vi "GetDVR.vi"(8 "error in (no error)":errorcluster, 11 "Menu in":refnum<class "Menu.lvclass">) -> (0 "error out":errorcluster, 2 "DVR":refnum<data-value>, 3 "Menu out":refnum<class "Menu.lvclass">)   [LabVIEW 2021, in "Menu.lvlib" / "Menu.lvclass"]
uses:
  Menu.lvclass
  Menu.lvclass/Menu.ctl
  MenuItems.ctl
  Data.ctl
  <vilib>/Utility/miscctls.llb/LVMenuShortCut.ctl
  MenuSelection.ctl
  TD_CloseEvent.ctl
  Picture2D/src/Color/Color.lvclass
  MenuColors.ctl
  Picture2D/src/Picture/Image.lvclass
  Picture2D/src/Font/Font.lvclass
  SubMenuIcon.ctl
  Picture2D/src/Picture2D/Picture2D.lvclass
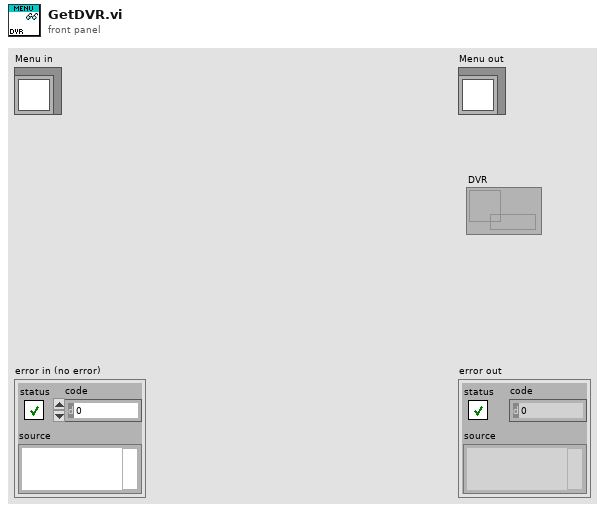
[diagram p1: front panel]
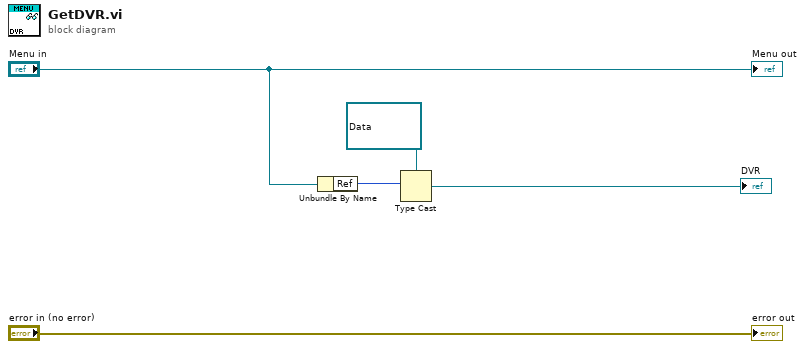
[diagram p0: block diagram]
diagram:
  n1 = Unbundle By Name("Menu in") -> ("Ref"=w1:u64)
  n2 = Type Cast(type=refnum<data-value> refnum ("data value reference"), x=w1) -> (*(type *) &x=→"DVR":refnum<data-value>)
  "error out" <- "error in (no error)"
  "Menu out" <- "Menu in"
